vi "Config Close Inlet Outlet Step.vi"(0 "FPGA API in":refnum<class "FPGA API Concrete.lvclass">, 5 "sp [mA]":dbl, 11 "error in (no error)":errorcluster, 13 "Enum":T1(ring)) -> (4 "FPGA API out":refnum<class "FPGA API Concrete.lvclass">, 6 "sp [mA] dub":dbl, 15 "error out":errorcluster)   [LabVIEW 2019, in "FPGA API Concrete.lvclass"]
uses:
  FPGA API Concrete.lvclass
  FPGA API Concrete.lvclass/FPGA API Concrete.ctl
  <vilib>/Utility/error.llb/Error Cluster From Error Code.vi
  <vilib>/rvi/errors/niLvFpgaAdjustHostInterfaceError.vi
  <vilib>/rvi/interface/nirviReadWriteControl/nirviReadWriteControl.xnode
  FPGA Ref.ctl
  NiFpgaLv.dll
  <vilib>/rvi/interface/Simulation/niFpgaSimulationCallBeginRW.vi
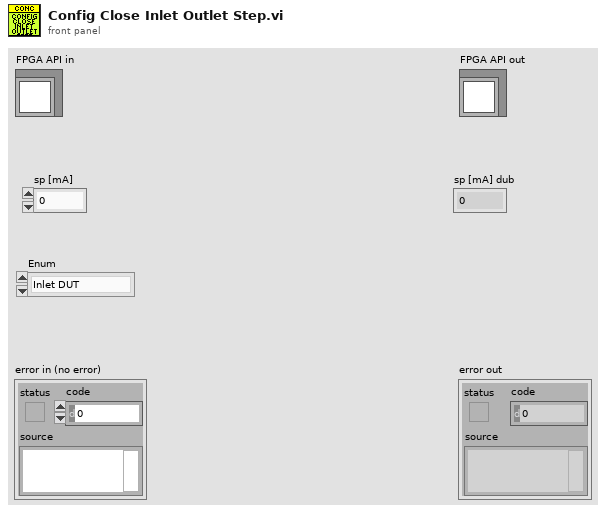
[diagram p1: front panel]
types:
  T1 = enum16{"Inlet DUT", "Outlet DUT", "StepDrive DUT", "Inlet Chamber", "Outlet Chamber", "StepDrive Chamber"}
  T2 = typedef "FPGA API Concrete.lvclass/FPGA Ref.ctl" = refnum<k20>
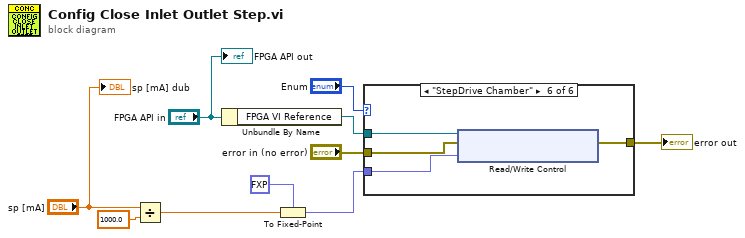
[diagram p0: block diagram]
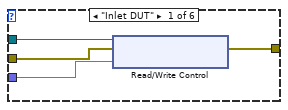
[diagram p2: hidden frame]
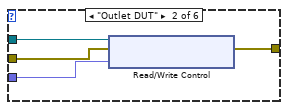
[diagram p3: hidden frame]
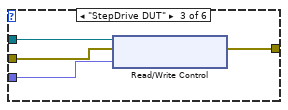
[diagram p4: hidden frame]
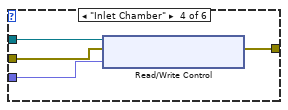
[diagram p5: hidden frame]
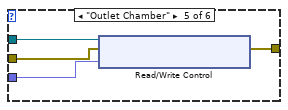
[diagram p6: hidden frame]
diagram:
  n1 = Divide(x="sp [mA]", y=1000.0) -> (x/y=w3:dbl)
  n2 = Unbundle By Name("FPGA API in") -> ("FPGA VI Reference"=w9:T2)
  n3 = To Fixed-Point(fixed-point type=fxp<+/-,21,-4> 0.0 ("SP Close Inlet"), number=w3) -> (fixed-point=w4:fxp<+/-,21,-4>)
  n4 = case shown="\"StepDrive Chamber\"" "Enum" {
    tunnel: w9 -> [w14 w18 w22 w26 w30 w34]
    tunnel: "error in (no error)" -> [w13 w17 w21 w25 w29 w33]
    tunnel: [w12 w16 w20 w24 w28 w32] -> w7
    tunnel: w4 -> [w11 w15 w19 w23 w27 w31]
    frame "Inlet DUT" {
      n5 = xnode "Read/Write Control"("FPGA VI Reference In"=w14, "error in"=w13, "SP Close Inlet DUT"=w11) -> ("error out"=w12:errorcluster)  [unwired: 1 out]
    }
    frame "Outlet DUT" {
      n6 = xnode "Read/Write Control"("FPGA VI Reference In"=w18, "error in"=w17, "SP Close Outlet DUT"=w15) -> ("error out"=w16:errorcluster)  [unwired: 1 out]
    }
    frame "StepDrive DUT" {
      n7 = xnode "Read/Write Control"("FPGA VI Reference In"=w22, "error in"=w21, "SP Stop Drive DUT"=w19) -> ("error out"=w20:errorcluster)  [unwired: 1 out]
    }
    frame "Inlet Chamber" {
      n8 = xnode "Read/Write Control"("FPGA VI Reference In"=w26, "error in"=w25, "SP Close Inlet Chamber"=w23) -> ("error out"=w24:errorcluster)  [unwired: 1 out]
    }
    frame "Outlet Chamber" {
      n9 = xnode "Read/Write Control"("FPGA VI Reference In"=w30, "error in"=w29, "SP Close Outlet Chamber"=w27) -> ("error out"=w28:errorcluster)  [unwired: 1 out]
    }
    frame "StepDrive Chamber" {
      n10 = xnode "Read/Write Control"("FPGA VI Reference In"=w34, "error in"=w33, "SP Stop Drive Chamber"=w31) -> ("error out"=w32:errorcluster)  [unwired: 1 out]
    }
  }
  "error out" <- w7
  "FPGA API out" <- "FPGA API in"
  "sp [mA] dub" <- "sp [mA]"
